vi "TextSynapses.vi"() -> ()   [LabVIEW 2016]
uses:
  Controls/Type of Neuron.ctl
  Cerebellum/Cerebellum.lvclass
  AER/AER.lvclass
panel:
  out "GOGC idx":i32[](array[numeric])
  out "W":dbl[](array[numeric])
  out "No Pre":i32[](array[numeric])
  out "Pre IDs":i32[](array[numeric])
  out "PFPC idx":i32[](array[numeric])
  out "No N":i32[](array[numeric])
  out "PCBA idx":i32[](array[numeric])
  out "BAGO idx":i32[](array[numeric])
  out "Neurons":string[](array[string])
  out "Array":string[](array[string])
  out "Synapses":string[](array[string])
  out "*(type *) &x":T1
  in  "Type of Neuron":T1
  out "Post Neurons":string[](array[string])
  in  "Right Hemis":path
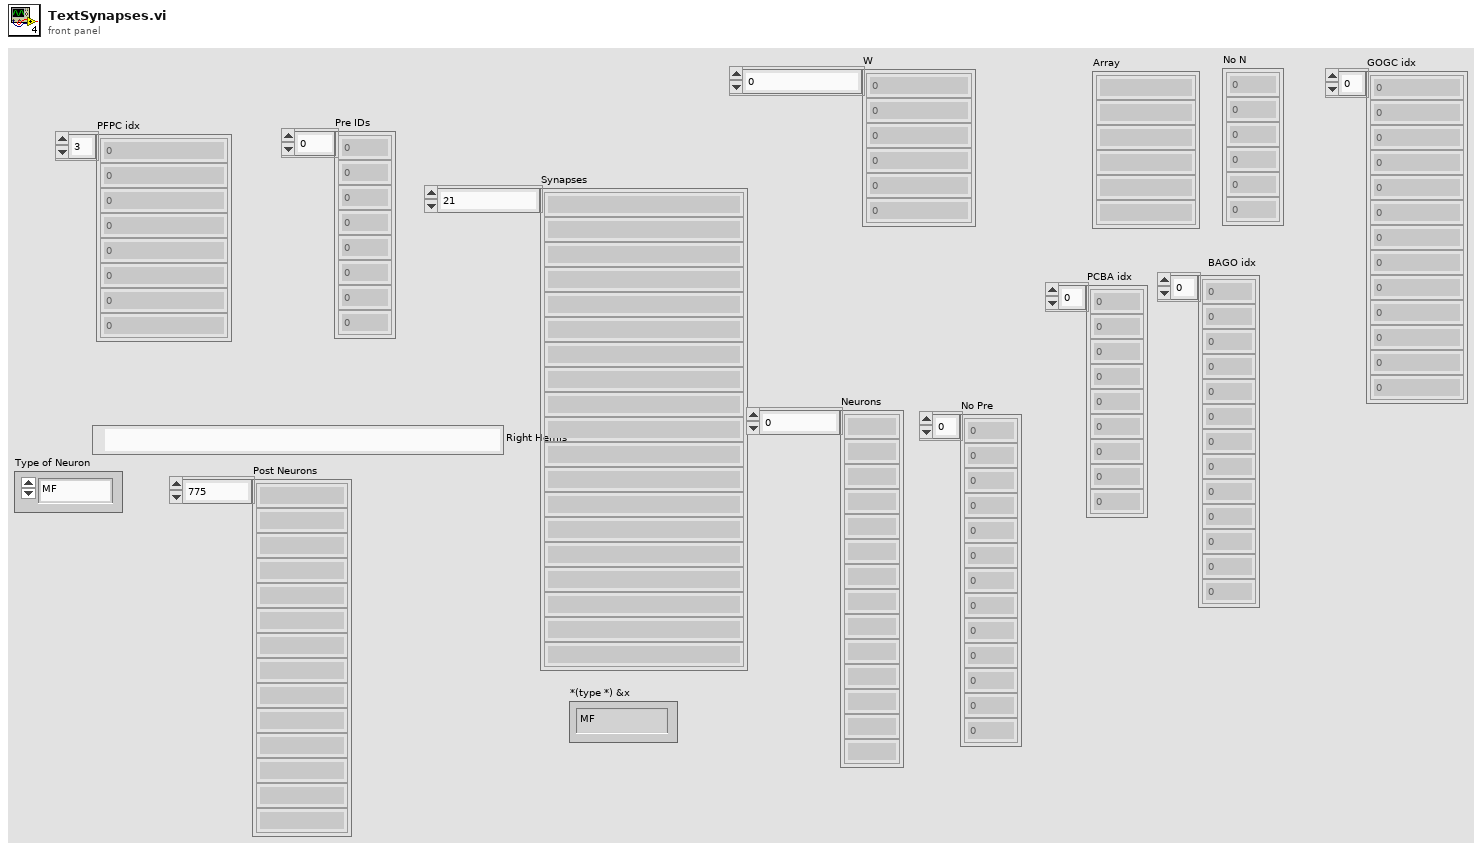
[diagram p1: front panel]
types:
  T1 = typedef "Type of Neuron.ctl" = enum16{"MF", "BA", "GO", "GC", "PC", "LU", "Glia (Dummy)"}
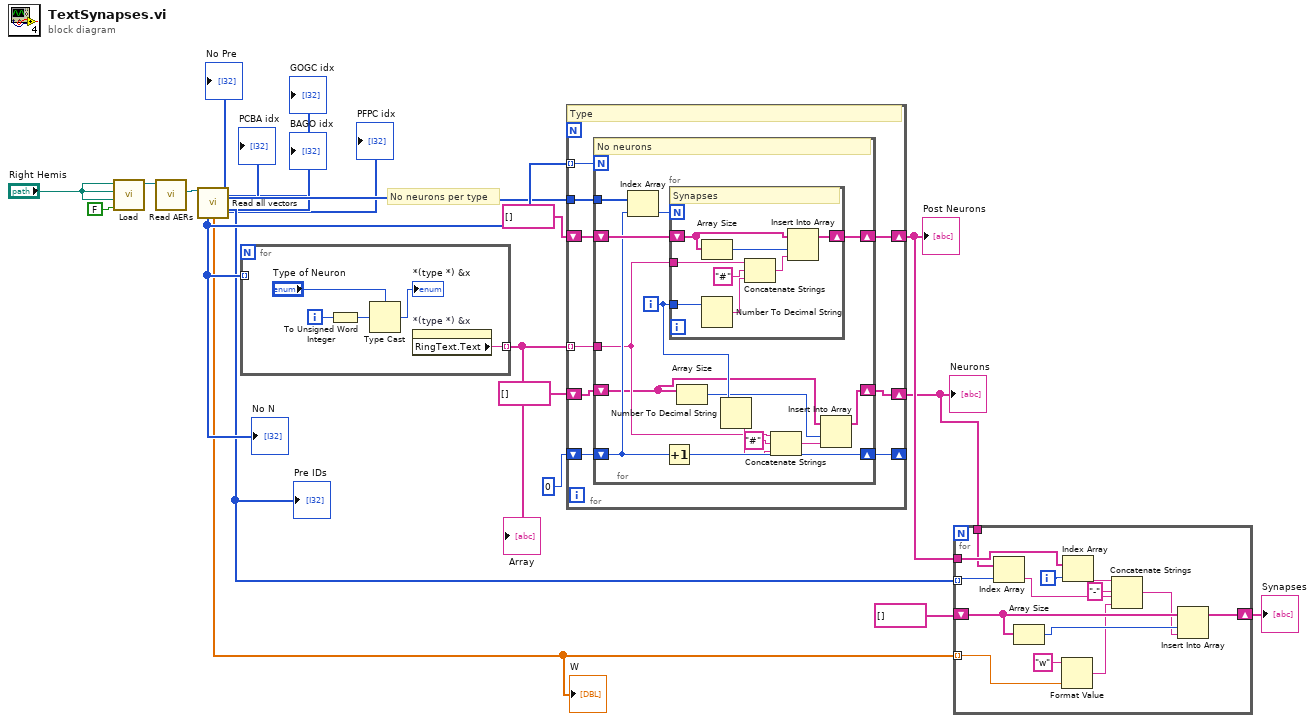
[diagram p0: block diagram]
diagram:
  # "No neurons per type"
  n1 = call "Load.vi"("Trained?"=FALSE, "Trained Path"="Right Hemis", "Left Hem Path"="Right Hemis", "Right Hem Path"="Right Hemis") -> ("Cerebellum out"=w19:refnum<class "Cerebellum.lvclass">)  [unwired: 7 in]
  n2 = call-dynamic "Read AERs.vi"("Cerebellum in"=w19) -> ("AER Left"=w18:refnum<class "AER.lvclass">)  [unwired: 7 in, 3 out]
  n3 = call-dynamic "Read all vectors.vi"("AER in"=w18) -> ("GOGC idx"=→"GOGC idx":i32[], "PCBA idx"=→"PCBA idx":i32[], "No Pre"=w13:i32[], "BAGO idx"=→"BAGO idx":i32[], "Pre IDs"=w11:i32[], "No N"=w14:i32[], "W"=w2:dbl[], "PFPC idx"=→"PFPC idx":i32[])  [unwired: 4 in, 3 out]
  "No N" <- w14
  "Pre IDs" <- w11
  "No Pre" <- w13
  "W" <- w2
  n4 = for {
    tunnel: w14 -> [_] mode=indexing
    tunnel: [w21] -> w15 mode=indexing
    i -> [w24]
    n5 = To Unsigned Word Integer(number=w24) -> (unsigned 16bit integer=w25:u16)
    n6 = Type Cast(type="Type of Neuron", x=w25) -> (*(type *) &x=→"*(type *) &x":T1)
    n7 = property on="*(type *) &x" class="Enum (strict)"() -> ("RingText.Text"=w21:string)  [unwired: 2 in, 2 out]
  }
  "Array" <- w15
  n8 = for {
    shift-right: [w34] -> w10
    shift-left: string[] [] -> [w33]
    tunnel: w15 -> [w32] mode=indexing
    tunnel: w14 -> [w31] mode=indexing
    tunnel: w13 -> [w29]
    shift-right: [w28] -> _
    shift-left: 0 -> [w30]
    shift-right: [w26] -> w6
    shift-left: string[] [] -> [w27]
    # "Type"
    n9 = for {
      N: w31 -> [_]
      tunnel: w32 -> [w39]
      shift-right: [w48] -> w34
      shift-left: w33 -> [w47]
      shift-right: [w46] -> w28
      shift-left: w30 -> [w44]
      tunnel: w29 -> [w45]
      shift-right: [w37] -> w26
      shift-left: w27 -> [w38]
      i -> [w42]
      # "No neurons"
      n10 = Index Array(array=w45, index=w44) -> (element=w43:i32)
      n11 = Increment(x=w44) -> (x+1=w46:i32)
      n12 = for {
        N: w43 -> [_]
        tunnel: w39 -> [w56]
        tunnel: w42 -> [w49]
        shift-right: [w52] -> w48
        shift-left: w47 -> [w51]
        # "Synapses"
        n13 = Array Size(array=w51) -> (size(s)=w50:i32)
        n14 = Number To Decimal String(number=w49) -> (decimal integer string=w55:string)  [unwired: 1 in]
        n15 = Concatenate Strings(w56, "#" ("string"), w55) -> (w53:string)
        n16 = Insert Into Array(array=w51, index=w50, new element=w53) -> (w52:string[])
      }
      n17 = Array Size(array=w38) -> (size(s)=w35:i32)
      n18 = Number To Decimal String(number=w42) -> (decimal integer string=w40:string)  [unwired: 1 in]
      n19 = Concatenate Strings(w39, "#" ("string"), w40) -> (w36:string)
      n20 = Insert Into Array(array=w38, index=w35, new element=w36) -> (w37:string[])
    }
  }
  "Post Neurons" <- w10
  "Neurons" <- w6
  n21 = for {
    tunnel: w11 -> [w70] mode=indexing
    tunnel: w10 -> [w66]
    shift-right: [w69] -> w8
    shift-left: string[] [] -> [w68]
    tunnel: w6 -> [w60]
    tunnel: w2 -> [w59] mode=indexing
    i -> [w65]
    n22 = Index Array(array=w60, index=w70) -> (element=w63:string)
    n23 = Array Size(array=w68) -> (size(s)=w67:i32)
    n24 = Format Value(string ("")="w", value (0)=w59) -> (output string=w58:string)  [unwired: 1 in]
    n25 = Index Array(array=w66, index=w65) -> (element=w64:string)
    n26 = Concatenate Strings(w64, "-" ("string"), w63, w58) -> (w61:string)
    n27 = Insert Into Array(array=w68, index=w67, new element=w61) -> (w69:string[])
  }
  "Synapses" <- w8
